vi "Get or Set MICS ID.vi"() -> (8 "Target":u32 format="%x", 15 "error out":errorcluster)   [LabVIEW 2010]
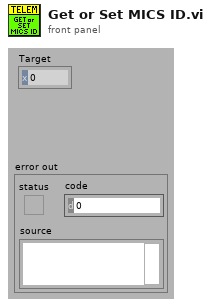
[diagram p1: front panel]
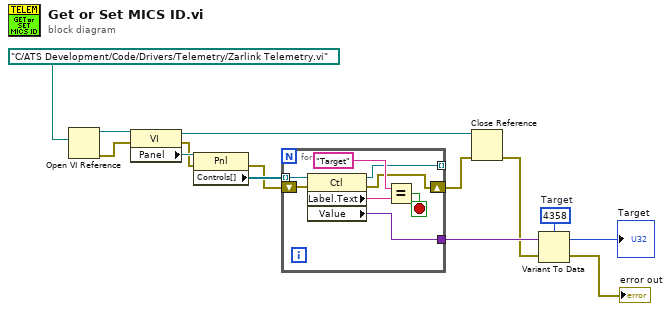
[diagram p0: block diagram]
diagram:
  w9 = u32 4358  # Target
  n1 = Open VI Reference(vi path=path "C:/ATS Development/Code/Drivers/Telemetry/Zarlink Telemetry.vi") -> (vi reference=w13:refnum<vi>, error out=w8:errorcluster)  [unwired: 5 in]
  n2 = property class="VI"(reference=w13, error in=w8) -> (reference out=w5:refnum<vi>, error out=w7:errorcluster, "Panel"=w12:refnum<vi>)
  n3 = property class="Pnl"(reference=w12, error in=w7) -> (error out=w6:errorcluster, "Controls[]"=w11:refnum<vi>[])  [unwired: 1 out]
  n4 = for {
    tunnel: w11 -> [w22] mode=indexing
    tunnel: [w21] -> w10
    shift-right: [w16] -> w4
    shift-left: w6 -> [w17]
    tunnel: [w15] -> _ mode=indexing
    stop <- w18 stop-if-true
    n5 = property class="Ctl"(reference=w22, error in=w17) -> (reference out=w15:refnum<vi>, error out=w16:errorcluster, "Label.Text"=w20:string, "Value"=w21:variant)
    n6 = Equal?(x="Target", y=w20) -> (x = y?=w18:bool)
  }
  n7 = Close Reference(reference=w5, error in (no error)=w4) -> (error out=w3:errorcluster)
  n8 = Variant To Data(error in=w3, Variant=w10, type=w9) -> (error out=→"error out":errorcluster, data=→"Target":u32)
